vi "AngleCorrection.vi"(4 "error in (no error)":errorcluster, 5 "TQGT":dbl[][](array[numeric])=[[-0.19101335575986092, -0.34474485039545594, -1.5808796689236986, -1.4329189178456425, 1.5166090092694082, 2.5485830374067953, -0.013484645322793008, -0.023218546346275737, 2.169326934039207], [4.8525463379547915e-05, 4.852385087889624e-05, 4.8847046573106735e-05, 4.835021438987554e-05, 4.84572062328829e-05, 4.909071065182245e-05, 4.6173748208842695e-05, 4.741257527869802e-05, 4.8633052093613115e-05], [0.15671932711808712, 0.35746595480793153, 0.014271561106869229, -0.02134803746821957, 0.039922199505364936, -0.009520900994179913, 0.0058362142404053225, 0.0071152104537498435, 0.02061179434094221], [2.4361385780568154, 0.8004545178296676, 2.453197893902325, 2.784014963639963, 2.971385034348702, 0.922978502998221, 0.14614862452661326, 3.1147864039841893, 0.28335828262986945], [9.888338299032878e-07, 2.097476055245101e-06, 6.189776896709198e-06, 4.448855607036343e-06, 6.887483856163851e-05, 0.00010163964796598845, 0.00011751108093782255, 0.00013310393450979466, 0.000110328053960891]], 6 "Psi":dbl, 7 "Data Before TCT":T2) -> (0 "error out":errorcluster, 3 "Data after TCT":T1)   [LabVIEW 2017, in "SignalConverson.lvlib"]
uses:
  SignalConverson.lvlib
  Data Before Angle Compensation.ctl
  Angle compensated data.ctl
panel:
  in  "Vx Yy correction?":bool=TRUE
  in  "As Gain (1) or Offset (0)":bool=TRUE
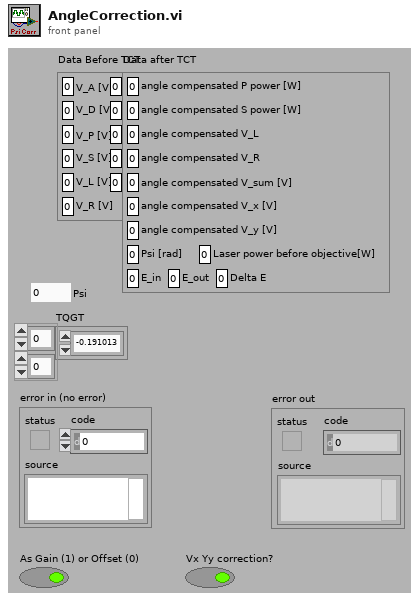
[diagram p1: front panel]
types:
  T1 = typedef "SignalConverson.lvlib/Angle compensated data.ctl" = cluster{"angle compensated P power [W]":dbl, "angle compensated S power [W]":dbl, "angle compensated V_L":dbl, "angle compensated V_R":dbl, "angle compensated V_sum [V]":dbl, "angle compensated V_x [V]":dbl, "angle compensated V_y [V]":dbl, "Psi [rad]":dbl, "Laser power before objective[W]":dbl, "E_in":dbl, "E_out":dbl, "Delta E":dbl}
  T2 = typedef "SignalConverson.lvlib/Data Before Angle Compensation.ctl" = cluster{"V_A [V]":dbl, "V_D [V]":dbl, "V_P [V]":dbl, "V_S [V]":dbl, "V_L [V]":dbl, "V_R [V]":dbl, "V_sum [V]":dbl, "V_x [V]":dbl, "V_y [V]":dbl, "P power [mW]":dbl, "S power [mW]":dbl}
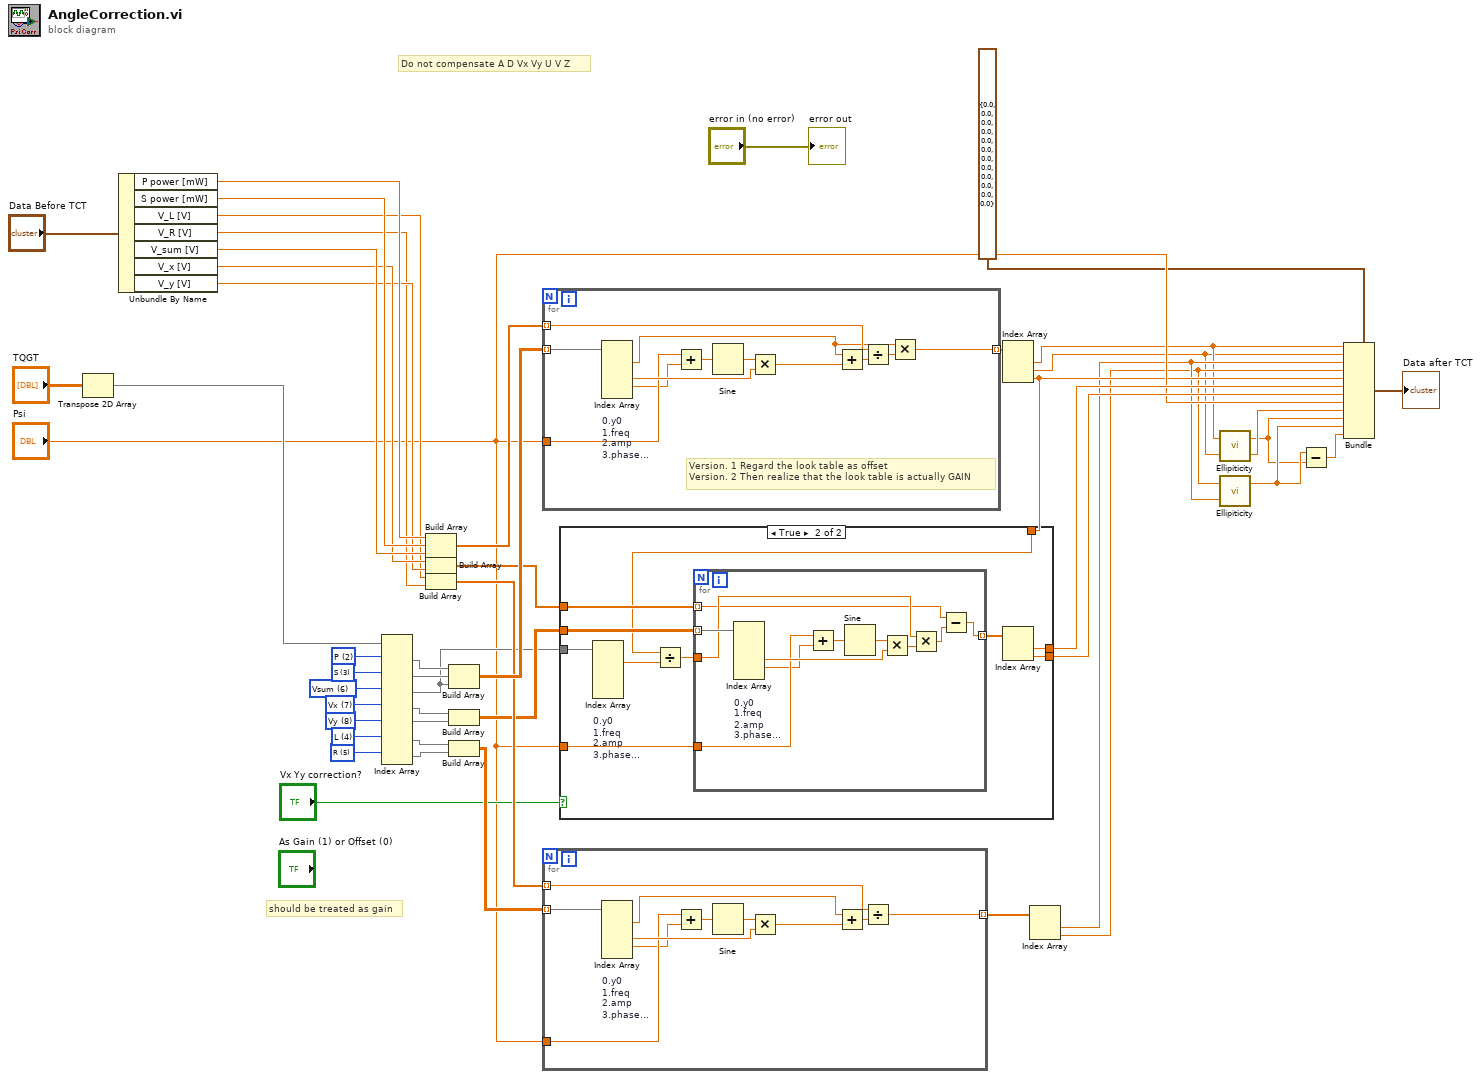
[diagram p0: block diagram]
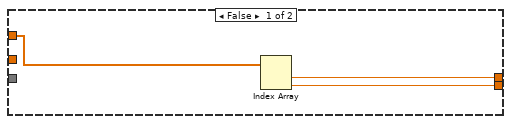
[diagram p2: hidden frame]
diagram:
  w32 = 8 items=["A", "D", "P", "S", "L", "R", "Vsum", "Vx", "Vy", "Piezo U", "Piezo V", "Piezo Z"] ("Channel 3")
  w33 = 7 items=["A", "D", "P", "S", "L", "R", "Vsum", "Vx", "Vy", "Piezo U", "Piezo V", "Piezo Z"] ("Channel 3")
  w43 = 6 items=["A", "D", "P", "S", "L", "R", "Vsum", "Vx", "Vy", "Piezo U", "Piezo V", "Piezo Z"] ("Channel 3")
  w44 = 3 items=["A", "D", "P", "S", "L", "R", "Vsum", "Vx", "Vy", "Piezo U", "Piezo V", "Piezo Z"] ("Channel 3")
  w45 = 2 items=["A", "D", "P", "S", "L", "R", "Vsum", "Vx", "Vy", "Piezo U", "Piezo V", "Piezo Z"] ("Channel 3")
  w35 = 5 items=["A", "D", "P", "S", "L", "R", "Vsum", "Vx", "Vy", "Piezo U", "Piezo V", "Piezo Z"] ("Channel 3")
  w34 = 4 items=["A", "D", "P", "S", "L", "R", "Vsum", "Vx", "Vy", "Piezo U", "Piezo V", "Piezo Z"] ("Channel 3")
  # "should be treated as gain"
  # "Do not compensate A D Vx Vy U V Z"
  n1 = Transpose 2D Array(2D array="TQGT") -> (transposed array=w46:dbl[][])
  n2 = Unbundle By Name("Data Before TCT") -> ("P power [mW]"=w21:dbl, "S power [mW]"=w20:dbl, "V_L [V]"=w16:dbl, "V_R [V]"=w15:dbl, "V_sum [V]"=w19:dbl, "V_x [V]"=w18:dbl, "V_y [V]"=w17:dbl)
  n3 = Index Array(array=w46, index (row) #1=w45, index (row) #2=w44, index (row) #3=w43, index (row) #4=w33, index (row) #5=w32, index (row) #6=w34, index (row) #7=w35) -> (element #1=w42:dbl[], element #2=w41:dbl[], element #3=w25:dbl[], element #4=w29:dbl[], element #5=w28:dbl[], element #6=w31:dbl[], element #7=w30:dbl[])  [unwired: 7 in]
  n4 = Build Array(w21, w20, w19) -> (w40:dbl[])
  n5 = Build Array(w18, w17) -> (w26:dbl[])
  n6 = Build Array(w16, w15) -> (w37:dbl[])
  n7 = Build Array(w42, w41, w25) -> (w39:dbl[][])
  n8 = Build Array(w29, w28) -> (w27:dbl[][])
  n9 = Build Array(w31, w30) -> (w36:dbl[][])
  n10 = for {
    tunnel: "Psi" -> [w58]
    tunnel: w40 -> [w55] mode=indexing
    tunnel: [w51] -> w38 mode=indexing
    tunnel: w39 -> [w54] mode=indexing
    # "Version. 1 Regard the look table as offset\nVersion. 2 Then realize that the look table is actually GAIN"
    n11 = Index Array "0.y0\n1.freq\n2.amp\n3.phase\n4.residue"(array=w54) -> (element #1=w52:dbl, element #3=w59:dbl, element #4=w57:dbl)  [unwired: 5 in, 2 out]
    n12 = Add(x=w58, y=w57) -> (x+y=w56:dbl)
    n13 = Sine(x=w56) -> (sin(x)=w60:dbl)
    n14 = Multiply(x=w60, y=w59) -> (x*y=w53:dbl)
    n15 = Add(x=w52, y=w53) -> (x+y=w50:dbl)
    n16 = Divide(x=w55, y=w50) -> (x/y=w49:dbl)
    n17 = Multiply(x=w52, y=w49) -> (x*y=w51:dbl)
  }
  n18 = for {
    tunnel: "Psi" -> [w69]
    tunnel: w37 -> [w66] mode=indexing
    tunnel: [w61] -> w23 mode=indexing
    tunnel: w36 -> [w65] mode=indexing
    n19 = Index Array "0.y0\n1.freq\n2.amp\n3.phase\n4.residue"(array=w65) -> (element #1=w63:dbl, element #3=w70:dbl, element #4=w68:dbl)  [unwired: 5 in, 2 out]
    n20 = Add(x=w69, y=w68) -> (x+y=w67:dbl)
    n21 = Sine(x=w67) -> (sin(x)=w71:dbl)
    n22 = Multiply(x=w71, y=w70) -> (x*y=w64:dbl)
    n23 = Add(x=w63, y=w64) -> (x+y=w62:dbl)
    n24 = Divide(x=w66, y=w62) -> (x/y=w61:dbl)
  }
  n25 = Index Array(array=w38) -> (element #1=w4:dbl, element #2=w3:dbl, element #3=w9:dbl)  [unwired: 3 in]
  n26 = case shown="True" "Vx Yy correction?" {
    tunnel: w27 -> [_ w84]
    tunnel: "Psi" -> [_ w83]
    tunnel: w26 -> [w74 w82]
    tunnel: w25 -> [_ w80]
    tunnel: w9 -> [_ w78]
    tunnel: [w73 w76] -> w14
    tunnel: [w72 w75] -> w13
    frame False {
      n27 = Index Array(array=w74) -> (element #1=w73:dbl, element #2=w72:dbl)  [unwired: 2 in]
    }
    frame True {
      n28 = Index Array "0.y0\n1.freq\n2.amp\n3.phase\n4.residue"(array=w80) -> (element #1=w79:dbl)  [unwired: 5 in, 4 out]
      n29 = Divide(x=w78, y=w79) -> (x/y=w77:dbl)
      n30 = for {
        tunnel: w83 -> [w93]
        tunnel: w82 -> [w85] mode=indexing
        tunnel: [w86] -> w81 mode=indexing
        tunnel: w84 -> [w90] mode=indexing
        tunnel: w77 -> [w89]
        n31 = Index Array "0.y0\n1.freq\n2.amp\n3.phase\n4.residue"(array=w90) -> (element #3=w94:dbl, element #4=w92:dbl)  [unwired: 5 in, 3 out]
        n32 = Add(x=w93, y=w92) -> (x+y=w91:dbl)
        n33 = Sine(x=w91) -> (sin(x)=w95:dbl)
        n34 = Multiply(x=w95, y=w94) -> (x*y=w88:dbl)
        n35 = Multiply(x=w89, y=w88) -> (x*y=w87:dbl)
        n36 = Subtract(x=w85, y=w87) -> (x-y=w86:dbl)
      }
      n37 = Index Array(array=w81) -> (element #1=w76:dbl, element #2=w75:dbl)  [unwired: 2 in]
    }
  }
  n38 = Index Array(array=w23) -> (element #1=w8:dbl, element #2=w7:dbl)  [unwired: 2 in]
  n39 = call "Ellipiticity.vi"("S"=w3, "P"=w4) -> ("P+S"=w2:dbl, "(P-S)/(P+S)"=w1:dbl)
  n40 = call "Ellipiticity.vi"("S"=w8, "P"=w7) -> ("(P-S)/(P+S)"=w5:dbl)  [unwired: 1 out]
  n41 = Subtract(x=w5, y=w1) -> (x-y=w6:dbl)
  n42 = Bundle(cluster=T1 {"angle compensated P power [W]"=0.0, "angle compensated S power [W]"=0.0, "angle compensated V_L"=0.0, "angle compensated V_R"=0.0, "angle compensated V_sum [V]"=0.0, "angle compensated V_x [V]"=0.0, "angle compensated V_y [V]"=0.0, "Psi [rad]"=0.0, "Laser power before objective[W]"=0.0, "E_in"=0.0, "E_out"=0.0, "Delta E"=0.0} ("Data after TCT"), "angle compensated P power [W]"=w4, "angle compensated S power [W]"=w3, "angle compensated V_L"=w8, "angle compensated V_R"=w7, "angle compensated V_sum [V]"=w9, "angle compensated V_x [V]"=w14, "angle compensated V_y [V]"=w13, "Psi [rad]"="Psi", "Laser power before objective[W]"=w2, "E_in"=w1, "E_out"=w5, "Delta E"=w6) -> (→"Data after TCT":T1)
  "error out" <- "error in (no error)"
